vi "4461.Trigger.vi"(8 "error in (no error)":errorcluster, 11 "Instrument.Lockin in":refnum<class "Instrument.Lockin.lvclass">) -> (0 "error out":errorcluster, 3 "Instrument.Lockin out":refnum<class "Instrument.Lockin.lvclass">)   [LabVIEW 2016, in "Instrument.Lockin.lvclass"]
uses:
  Instrument.Lockin.lvclass
  <resource>/objmgr/daqmx.rc
  Typedefs/DAQType-enum.ctl
  <vilib>/DAQmx/configure/trigger.llb/DAQmx Start Trigger (Digital Edge).vi
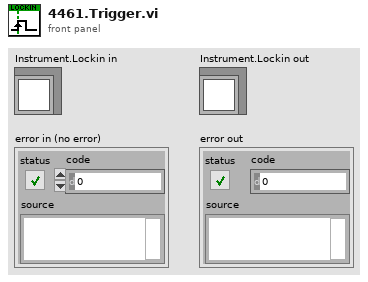
[diagram p1: front panel]
types:
  T1 = typedef "Instrument.Lockin.lvclass/DAQType-enum.ctl" = enum16{"None", "USB 4431", "PXI 446x"}
  T2 = cluster{"DAQ Type":T1, "master task":refnum<k21>, "RefClk.Src":tag, "SyncPulse.Src":tag, "Trigger.Src":tag, "SyncPulse.SyncTime":dbl}
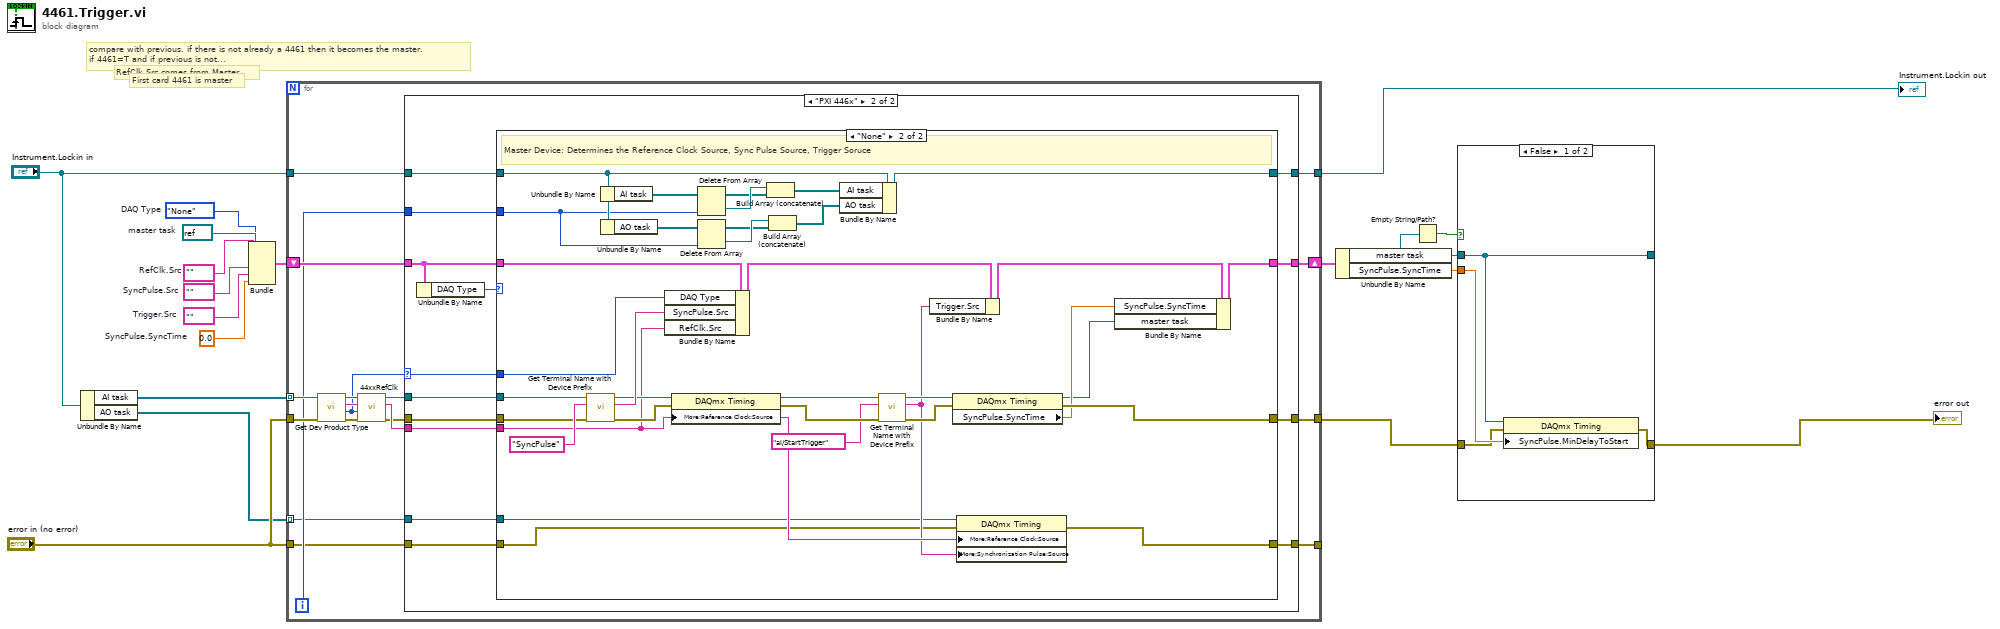
[diagram p0: block diagram]
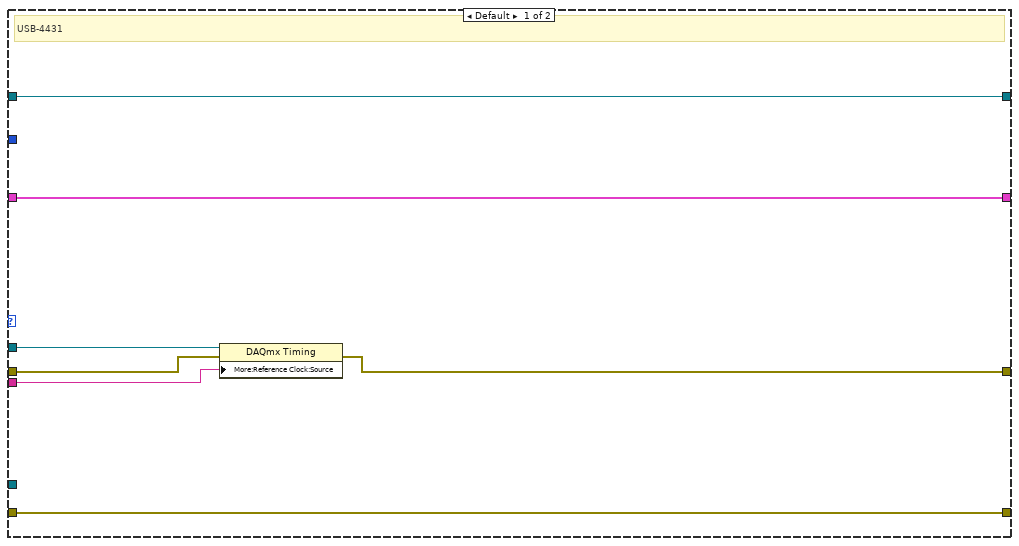
[diagram p2: hidden frame]
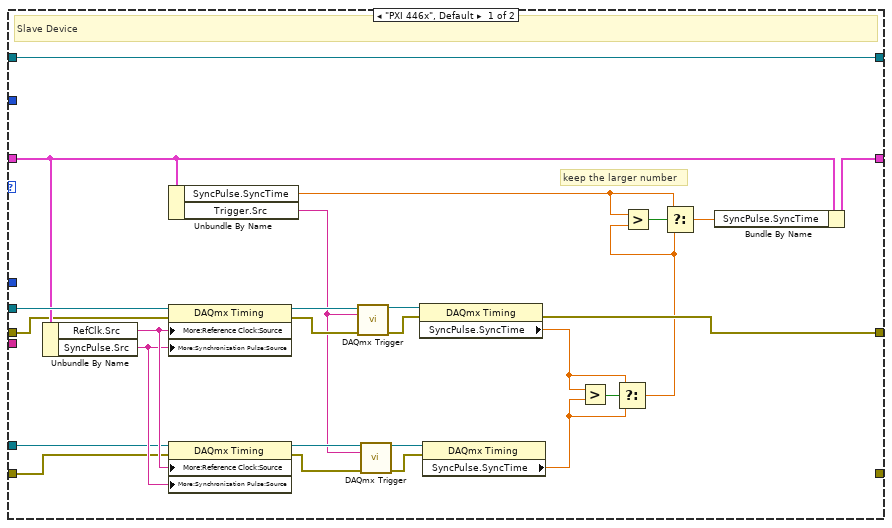
[diagram p3: hidden frame]
diagram:
  w12 = refnum<k21> refnum  # master task
  w10 = 0.0  # SyncPulse.SyncTime
  w9 = tag ""  # Trigger.Src
  w8 = tag ""  # SyncPulse.Src
  w7 = tag ""  # RefClk.Src
  w11 = DAQType-enum."None"  # DAQ Type
  # "RefClk.Src comes from Master"
  # "compare with previous. if there is not already a 4461 then it becomes the master. \nif 4461=T and if previous is not..."
  # "First card 4461 is master"
  n1 = Unbundle By Name("Instrument.Lockin in") -> ("AI task"=w3:refnum<k21>[], "AO task"=w1:refnum<k21>[])
  n2 = Bundle("DAQ Type"=w11, "master task"=w12, "RefClk.Src"=w7, "SyncPulse.Src"=w8, "Trigger.Src"=w9, "SyncPulse.SyncTime"=w10) -> (w6:T2)  [unwired: 1 in]
  n3 = for {
    tunnel: w3 -> [w36] mode=indexing
    tunnel: "error in (no error)" -> [w32]
    shift-right: [w27] -> w13
    shift-left: w6 -> [w30]
    tunnel: [w25] -> w17
    tunnel: "Instrument.Lockin in" -> [w24]
    tunnel: [w22] -> w4
    tunnel: [w21] -> _
    tunnel: "error in (no error)" -> [w20]
    tunnel: w1 -> [w19] mode=indexing
    i -> [w23]
    n4 = call "Get Dev Product Type.vi"("error in (no error)"=w32, "Refnum in"=w36) -> ("error out"=w35:errorcluster, "DAQ Type"=w31:T1, "ActiveDev"=w34:tag, "Refnum out"=w33:refnum<k21>)  [unwired: 6 in]
    n5 = call "44xxRefClk.vi"("error in (no error)"=w35, "DAQ Type"=w31, "ActiveDev"=w34, "Refnum in"=w33) -> ("error out"=w26:errorcluster, "RefClk.Src"=w28:tag, "Refnum out"=w29:refnum<k21>)  [unwired: 5 in]
    n6 = case shown="\"PXI 446x\"" w31 {
      selector: w31 -> [_ w54]
      tunnel: w30 -> [w43 w55]
      tunnel: w29 -> [w42 w57]
      tunnel: w28 -> [w41 w56]
      tunnel: [w43 w53] -> w27
      tunnel: w26 -> [w40 w52]
      tunnel: [w39 w51] -> w25
      tunnel: w24 -> [w38 w49]
      tunnel: w23 -> [_ w48]
      tunnel: [w38 w47] -> w22
      tunnel: [w37 w44] -> w21
      tunnel: w20 -> [w37 w46]
      tunnel: w19 -> [_ w45]
      frame Default {
        # "USB-4431"
        n7 = property class="DAQmx Timing"(reference=w42, error in=w40, "More:Reference Clock:Source"=w41) -> (error out=w39:errorcluster)  [unwired: 1 out]
      }
      frame "PXI 446x" {
        n8 = Unbundle By Name(w55) -> ("DAQ Type"=w50:T1)
        n9 = case shown="\"None\"" w50 {
          tunnel: w57 -> [w83 w118]
          tunnel: w56 -> [_ w94]
          tunnel: w55 -> [w80 w117]
          tunnel: w54 -> [_ w116]
          tunnel: [w79 w105] -> w53
          tunnel: w52 -> [w61 w113]
          tunnel: [w75 w104] -> w51
          tunnel: w49 -> [w74 w89]
          tunnel: w48 -> [_ w88]
          tunnel: [w74 w95] -> w47
          tunnel: w46 -> [w60 w91]
          tunnel: w45 -> [w71 w92]
          tunnel: [_ w90] -> w44
          frame "PXI 446x", Default {
            # "keep the larger number"
            # "Slave Device"
            n10 = Unbundle By Name(w80) -> ("RefClk.Src"=w73:tag, "SyncPulse.Src"=w72:tag)
            n11 = Unbundle By Name(w80) -> ("SyncPulse.SyncTime"=w59:dbl, "Trigger.Src"=w67:tag)
            n12 = property class="DAQmx Timing"(reference=w83, error in=w61, "More:Reference Clock:Source"=w73, "More:Synchronization Pulse:Source"=w72) -> (reference out=w82:refnum<k21>, error out=w68:errorcluster)
            n13 = property class="DAQmx Timing"(reference=w71, error in=w60, "More:Reference Clock:Source"=w73, "More:Synchronization Pulse:Source"=w72) -> (reference out=w69:refnum<k21>, error out=w66:errorcluster)
            n14 = call-poly <vilib>:"DAQmx Trigger.vi"("task/channels in"=w82, "source"=w67, "error in"=w68) -> ("task out"=w81:refnum<k21>, "error out"=w77:errorcluster)  [unwired: 11 in]
            n15 = call-poly <vilib>:"DAQmx Trigger.vi"("task/channels in"=w69, "source"=w67, "error in"=w66) -> ("task out"=w70:refnum<k21>, "error out"=w65:errorcluster)  [unwired: 11 in]
            n16 = property class="DAQmx Timing"(reference=w81, error in=w77) -> (error out=w75:errorcluster, "SyncPulse.SyncTime"=w63:dbl)  [unwired: 1 out]
            n17 = property class="DAQmx Timing"(reference=w70, error in=w65) -> ("SyncPulse.SyncTime"=w62:dbl)  [unwired: 2 out]
            n18 = Greater?(x=w63, y=w62) -> (0:w64:bool)
            n19 = Select(t=w63, s=w64, f=w62) -> (s? t:f=w58:dbl)
            n20 = Greater?(x=w59, y=w58) -> (0:w76:bool)
            n21 = Select(t=w59, s=w76, f=w58) -> (s? t:f=w78:dbl)
            n22 = Bundle By Name(cluster=w80, "SyncPulse.SyncTime"=w78) -> (w79:T2)
          }
          frame "None" {
            # "Master Device: Determines the Reference Clock Source, Sync Pulse Source, Trigger Soruce"
            n23 = call "Get Terminal Name with Device Prefix.vi"("error in (no error)"=w113, "Local Terminal Name"="SyncPulse", "task/channels in"=w118) -> ("error out"=w112:errorcluster, "Terminal Name with Device Prefix"=w114:tag, "task out"=w101:refnum<k21>)  [unwired: 6 in]
            n24 = Unbundle By Name(w89) -> ("AI task"=w99:refnum<k21>[])
            n25 = Unbundle By Name(w89) -> ("AO task"=w87:refnum<k21>[])
            n26 = Bundle By Name(cluster=w117, "DAQ Type"=w116, "SyncPulse.Src"=w114, "RefClk.Src"=w94) -> (w108:T2)
            n27 = property class="DAQmx Timing"(reference=w101, error in=w112, "More:Reference Clock:Source"=w94) -> (reference out=w109:refnum<k21>, error out=w111:errorcluster)
            n28 = Delete From Array(array=w99, index=w88) -> (deleted portion=w98:refnum<k21>, array with subset deleted=w97:refnum<k21>[])  [unwired: 1 in]
            n29 = Delete From Array(array=w87, index=w88) -> (deleted portion=w86:refnum<k21>, array with subset deleted=w85:refnum<k21>[])  [unwired: 1 in]
            n30 = Build Array (concatenate)(w98, w97) -> (w96:refnum<k21>[])
            n31 = Build Array (concatenate)(w86, w85) -> (w84:refnum<k21>[])
            n32 = Bundle By Name(cluster=w89, "AI task"=w96, "AO task"=w84) -> (w95:refnum<class "Instrument.Lockin.lvclass">)
            n33 = call "Get Terminal Name with Device Prefix.vi"("error in (no error)"=w111, "Local Terminal Name"="ai/StartTrigger", "task/channels in"=w109) -> ("error out"=w106:errorcluster, "Terminal Name with Device Prefix"=w93:tag, "task out"=w107:refnum<k21>)  [unwired: 6 in]
            n34 = Bundle By Name(cluster=w108, "Trigger.Src"=w93) -> (w103:T2)
            n35 = property class="DAQmx Timing"(reference=w107, error in=w106) -> (reference out=w100:refnum<k21>, error out=w104:errorcluster, "SyncPulse.SyncTime"=w102:dbl)
            n36 = property class="DAQmx Timing"(reference=w92, error in=w91, "More:Reference Clock:Source"=w94, "More:Synchronization Pulse:Source"=w93) -> (error out=w90:errorcluster)  [unwired: 1 out]
            n37 = Bundle By Name(cluster=w103, "SyncPulse.SyncTime"=w102, "master task"=w100) -> (w105:T2)
          }
        }
      }
    }
  }
  "Instrument.Lockin out" <- w4
  n38 = Unbundle By Name(w13) -> ("master task"=w15:refnum<k21>, "SyncPulse.SyncTime"=w16:dbl)
  n39 = Empty String/Path?(string/path=w15) -> (empty?=w14:bool)
  n40 = case shown="False" w14 {
    tunnel: w15 -> [w119 w123]
    tunnel: w16 -> [w122 _]
    tunnel: w17 -> [w121 w124]
    tunnel: [w120 w124] -> w18
    tunnel: [w119 w123] -> _
    frame False {
      n41 = property class="DAQmx Timing"(reference=w119, error in=w121, "SyncPulse.MinDelayToStart"=w122) -> (error out=w120:errorcluster)  [unwired: 1 out]
    }
    frame True {
      # "If master task=empty, then no master devices were ever found (ie, all 4431s"
    }
  }
  "error out" <- w18
